vi "Calculate Desired States.vi"(8 "error in (no error)":errorcluster, 10 "Vessel In":refnum<class "Vessel.lvclass">, 11 "Altitude Guidance in":refnum<class "Altitude Guidance.lvclass">) -> (0 "error out":errorcluster, 2 "Vessel Out":refnum<class "Vessel.lvclass">, 3 "Altitude Guidance out":refnum<class "Altitude Guidance.lvclass">)   [LabVIEW 2014, in "Guidance Library.lvlib" / "Altitude Guidance.lvclass"]
uses:
  Altitude Guidance.lvclass
  ROV/Vessel.lvclass
  Supervisor/Supervisor.lvclass
panel:
  in  "PI_alt":dbl[](array[numeric])=[0.2, 0.0]
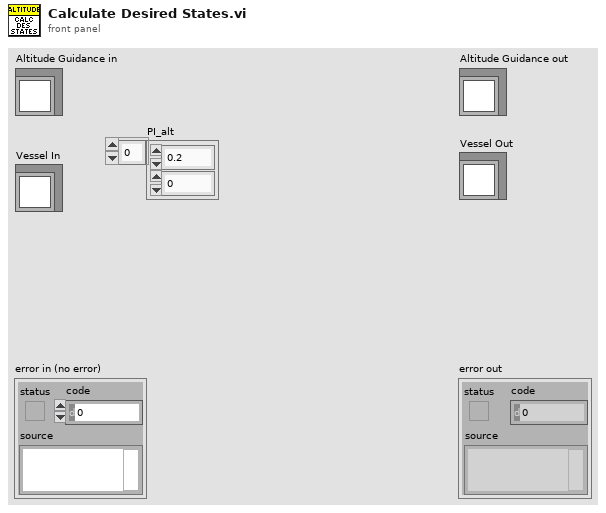
[diagram p1: front panel]
types:
  T1 = cluster{"Measured":cluster{"Eta":dbl[], "Nu":dbl[], "Eta Dot":dbl[], "Nu Dot":dbl[]}, "Estimated":cluster{"Eta":dbl[], "Nu":dbl[], "Eta Dot":dbl[], "Nu Dot":dbl[]}, "Desired":cluster{"Eta":dbl[], "Nu":dbl[], "Eta Dot":dbl[], "Nu Dot":dbl[]}, "Previous Desired":cluster{"Eta":dbl[], "Nu":dbl[], "Eta Dot":dbl[], "Nu Dot":dbl[]}, "tau":dbl[], "Altitude":cluster{"Measured":dbl, "Estimated":dbl, "Desired":dbl, "Previous Desired":dbl, "Approximated":dbl, "grad F":dbl[]}, "rpm":dbl[], "Attitude":cluster{"Theta Measured":dbl[], "Theta Estimated":dbl[], "Omega Measured":dbl[], "Omega Estimated":dbl[], "Gyro Bias":dbl[]}}
  T2 = cluster{"Use Integrator":bool, "Use FeedForward":bool, "Reset Reference Model":bool, "Desired Altitude":dbl}
  T3 = typedef "NI_Matrix.lvlib/RealMatrix.ctl" = dbl[][]
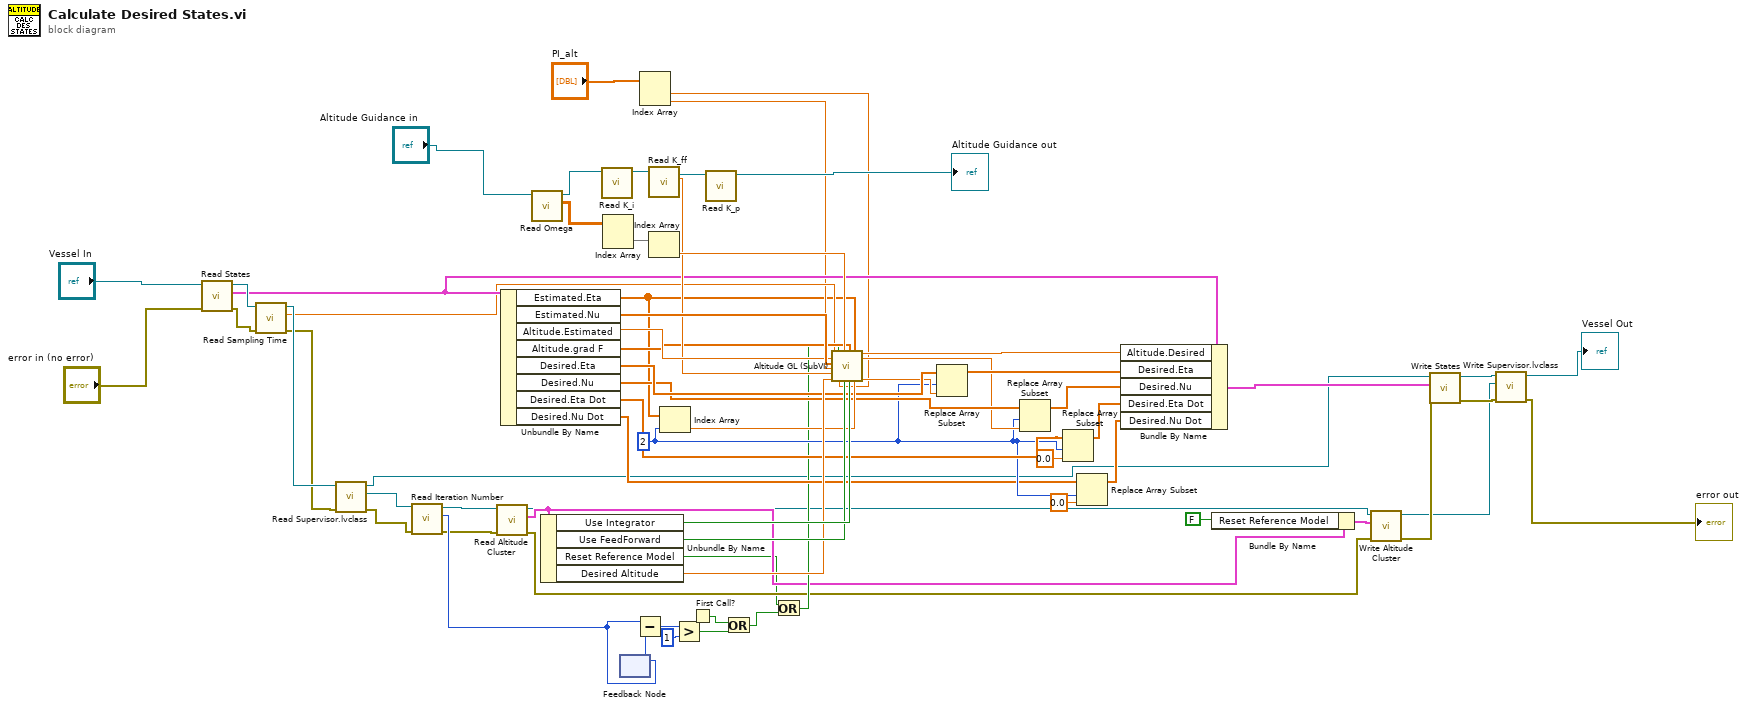
[diagram p0: block diagram]
diagram:
  w35 = 2 ("index")
  n1 = call-dynamic "Read States.vi"("error in (no error)"="error in (no error)", "Vessel in"="Vessel In") -> ("error out"=w20:errorcluster, "States"=w50:T1, "Vessel out"=w67:refnum<class "Vessel.lvclass">)  [unwired: 7 in]
  n2 = call-dynamic "Read Sampling Time.vi"("error in (no error)"=w20, "Vessel in"=w67) -> ("error out"=w19:errorcluster, "Sampling Time"=w43:dbl, "Vessel out"=w44:refnum<class "Vessel.lvclass">)  [unwired: 7 in]
  n3 = call "Read Supervisor.lvclass.vi"("error in (no error)"=w19, "Vessel in"=w44) -> ("error out"=w18:errorcluster, "Supervisor.lvclass"=w24:refnum<class "Supervisor.lvclass">, "Vessel out"=w8:refnum<class "Vessel.lvclass">)  [unwired: 7 in]
  n4 = call-dynamic "Read Iteration Number.vi"("error in (no error)"=w18, "Supervisor in"=w24) -> ("error out"=w17:errorcluster, "Iteration Number"=w22:i32, "Supervisor out"=w23:refnum<class "Supervisor.lvclass">)  [unwired: 7 in]
  n5 = call-dynamic "Read Altitude Cluster.vi"("error in (no error)"=w17, "Supervisor in"=w23) -> ("error out"=w13:errorcluster, "Altitude Cluster"=w14:T2, "Supervisor out"=w10:refnum<class "Supervisor.lvclass">)  [unwired: 7 in]
  n6 = Unbundle By Name(w50) -> ("Estimated.Eta"=w1:dbl[], "Estimated.Nu"=w62:dbl[], "Altitude.Estimated"=w61:dbl, "Altitude.grad F"=w55:dbl[], "Desired.Eta"=w47:dbl[], "Desired.Nu"=w42:dbl[], "Desired.Eta Dot"=w39:dbl[], "Desired.Nu Dot"=w34:dbl[])
  n7 = call-dynamic "Read Omega.vi"("Guidance in"="Altitude Guidance in") -> ("Omega"=w65:T3, "Guidance out"=w57:refnum<class "Altitude Guidance.lvclass">)  [unwired: 8 in, 1 out]
  n8 = Unbundle By Name(w14) -> ("Use Integrator"=w54:bool, "Use FeedForward"=w53:bool, "Reset Reference Model"=w9:bool, "Desired Altitude"=w52:dbl)
  n9 = call-dynamic "Read K_i.vi"("Altitude Guidance in"=w57) -> ("Altitude Guidance out"=w59:refnum<class "Altitude Guidance.lvclass">)  [unwired: 8 in, 2 out]
  n10 = Index Array(array=w65) -> (element=w64:dbl[])  [unwired: 2 in]
  n11 = feedback #1() -> (w29:i32)  [unwired: 1 in]
  n12 = feedback-in #1(w22) -> ()
  n13 = Subtract(x=w22, y=w29) -> (x-y=w28:i32)
  n14 = Index Array(array="PI_alt") -> (element #1=w31:dbl, element #2=w30:dbl)  [unwired: 2 in]
  n15 = call-dynamic "Read K_ff.vi"("Altitude Guidance in"=w59) -> ("K_ff"=w60:dbl, "Altitude Guidance out"=w58:refnum<class "Altitude Guidance.lvclass">)  [unwired: 8 in, 1 out]
  n16 = Index Array(array=w64) -> (element=w63:dbl)  [unwired: 1 in]
  n17 = Index Array(array=w1, index=w35) -> (element=w51:dbl)
  n18 = Greater?(x=w28, y=1) -> (0:w26:bool)
  n19 = First Call?() -> (First Call?: T/F=w25:bool)
  n20 = call-dynamic "Read K_p.vi"("Altitude Guidance in"=w58) -> ("Altitude Guidance out"=→"Altitude Guidance out":refnum<class "Altitude Guidance.lvclass">)  [unwired: 8 in, 2 out]
  n21 = Or(x=w25, y=w26) -> (x .or. y?=w16:bool)
  n22 = Or(x=w9, y=w16) -> (x .or. y?=w15:bool)
  n23 = call "Altitude GL (SubVI).vi"("dt"=w43, "a_hat"=w61, "nu_hat"=w62, "k_i alt"=w30, "k_ff alt"=w60, "des alt [m] in"=w52, "Boolean"=w15, "k_p alt"=w31, "omega alt"=w63, "ff on"=w53, "grad_F"=w55, "int on"=w54, "eta_hat"=w1, "depth_ic"=w51) -> ("a_des"=w49:dbl, "w_des"=w41:dbl, "d_des"=w46:dbl)  [unwired: 3 in]
  n24 = Replace Array Subset(array=w47, new element=w46, index=w35) -> (w48:dbl[])
  n25 = Replace Array Subset(array=w42, new element=w41, index=w35) -> (w40:dbl[])
  n26 = Replace Array Subset(array=w39, new element=0.0 ("new element/subarray"), index=w35) -> (w37:dbl[])
  n27 = Replace Array Subset(array=w34, new element=0.0 ("new element/subarray"), index=w35) -> (w33:dbl[])
  n28 = Bundle By Name(cluster=w50, "Altitude.Desired"=w49, "Desired.Eta"=w48, "Desired.Nu"=w40, "Desired.Eta Dot"=w37, "Desired.Nu Dot"=w33) -> (w45:T1)
  n29 = Bundle By Name(cluster=w14, "Reset Reference Model"=FALSE) -> (w11:T2)
  n30 = call-dynamic "Write Altitude Cluster.vi"("error in (no error)"=w13, "Altitude Cluster"=w11, "Supervisor in"=w10) -> ("error out"=w7:errorcluster, "Supervisor out"=w5:refnum<class "Supervisor.lvclass">)  [unwired: 7 in]
  n31 = call-dynamic "Write States.vi"("error in (no error)"=w7, "States"=w45, "Vessel in"=w8) -> ("error out"=w6:errorcluster, "Vessel out"=w4:refnum<class "Vessel.lvclass">)  [unwired: 7 in]
  n32 = call "Write Supervisor.lvclass.vi"("error in (no error)"=w6, "Supervisor.lvclass"=w5, "Vessel in"=w4) -> ("error out"=→"error out":errorcluster, "Vessel out"=→"Vessel Out":refnum<class "Vessel.lvclass">)  [unwired: 7 in]
